vi "Push Elements.vi"(8 "error in":errorcluster, 10 "elements":variant[](array[variant]), 11 "Buffer in":refnum<data-value>) -> (0 "error out":errorcluster, 3 "Buffer":refnum<data-value>)   [LabVIEW 2013, in "VariantBuffer.lvclass"]
doc: "This VI allows to input an array into the buffer. The location in the buffer is updated automatically.\n\nIf the input array is larger than the buffer then just take last elements of the input array and save them in the buffer. Also give a warning that this happened."
uses:
  VariantBuffer.lvclass
  VariantBuffer.lvclass/VariantBuffer.ctl
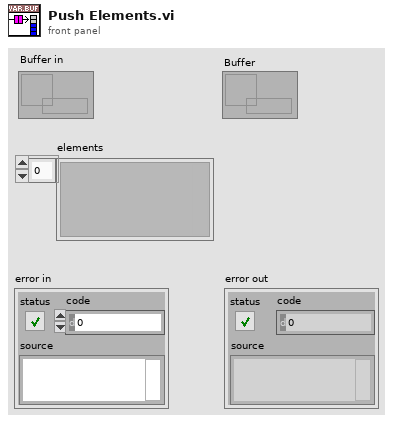
[diagram p1: front panel]
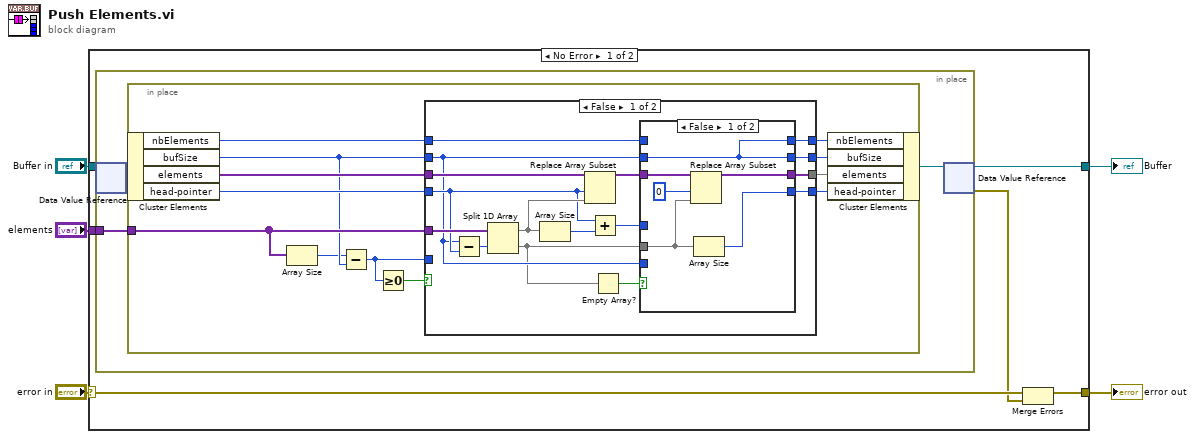
[diagram p0: block diagram]
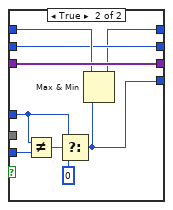
[diagram p2: hidden frame]
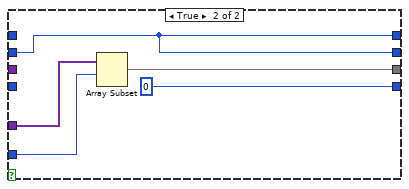
[diagram p3: hidden frame]
diagram:
  n1 = case shown="No Error" "error in" {
    selector: "error in" -> [w7 w64]
    tunnel: "Buffer in" -> [w11 w63]
    tunnel: [w10 w63] -> w4
    tunnel: [w9 w64] -> w3
    tunnel: "elements" -> [w8 _]
    frame No Error {
      n2 = in-place {
        in-place-border: w8 -> [w14]
        n3 = in-place-dvr #1(w11) -> (w13:refnum<class "VariantBuffer.lvclass">)  [unwired: 1 out]
        n4 = in-place {
          in-place-border: w14 -> [w22]
          n5 = in-place-cluster #2(w13) -> ("nbElements"=w19:i32, "bufSize"=w18:i32, "elements"=w26:variant[], "head-pointer"=w23:i32)
          n6 = Array Size(array=w22) -> (size(s)=w15:i32)
          n7 = Subtract(x=w15, y=w18) -> (x-y=w20:i32)
          n8 = Greater Or Equal To 0?(x=w20) -> (x >= 0?=w21:bool)
          n9 = case shown="False" w21 {
            tunnel: w26 -> [w42 _]
            tunnel: [w40 w60] -> w25
            tunnel: [w39 0 ("t")] -> w24
            tunnel: w23 -> [w33 _]
            tunnel: w22 -> [w34 w61]
            tunnel: w20 -> [_ w59]
            tunnel: w19 -> [w30 _]
            tunnel: w18 -> [w29 w58]
            tunnel: [w32 w58] -> w17
            tunnel: [w31 w58] -> w16
            frame False {
              n10 = Subtract(x=w29, y=w33) -> (x-y=w36:i32)
              n11 = Split 1D Array(array=w34, index=w36) -> (first subarray=w38:variant[], second subarray=w28:variant[])
              n12 = Array Size(array=w38) -> (size(s)=w37:i32)
              n13 = Replace Array Subset(array=w42, new element=w38, index=w33) -> (w41:variant[])
              n14 = Add(x=w33, y=w37) -> (x+y=w35:i32)
              n15 = Empty Array?(array=w28) -> (empty?=w27:bool)
              n16 = case shown="False" w27 {
                tunnel: w41 -> [w48 w57]
                tunnel: [w47 w57] -> w40
                tunnel: w28 -> [w44 _]
                tunnel: [w43 w49] -> w39
                tunnel: w35 -> [_ w53]
                tunnel: w29 -> [_ w54]
                tunnel: [w45 w51] -> w32
                tunnel: w29 -> [w45 w51]
                tunnel: [w45 w50] -> w31
                tunnel: w30 -> [_ w52]
                frame False {
                  n17 = Replace Array Subset(array=w48, new element=w44, index=0) -> (w47:variant[])
                  n18 = Array Size(array=w44) -> (size(s)=w43:i32)
                }
                frame True {
                  n19 = Not Equal?(x=w53, y=w54) -> (x != y?=w55:bool)
                  n20 = Select(t=w53, s=w55, f=0 ("t")) -> (s? t:f=w49:i32)
                  n21 = Max & Min(x=w52, y=w49) -> (max(x,y)=w50:i32)  [unwired: 1 out]
                }
              }
            }
            frame True {
              n22 = Array Subset(array=w61, index=w59) -> (w60:variant[])  [unwired: 1 in]
            }
          }
          n23 = in-place-cluster #2("nbElements"=w16, "bufSize"=w17, "elements"=w25, "head-pointer"=w24) -> (w12:refnum<class "VariantBuffer.lvclass">)
        }
        n24 = in-place-dvr #1(w12) -> (w10:refnum<data-value>, w6:errorcluster)
      }
      n25 = Merge Errors(w7, w6) -> (w9:errorcluster)
    }
    frame Error {
    }
  }
  "error out" <- w3
  "Buffer" <- w4
